vi "SpectrumIndex.vi"(9 "Freq":dbl=867920000.0 format="%#_13g", 11 "Spectrum":cluster{"f0":dbl, "df":dbl, "magnitude":dbl[]}) -> (1 "magnitude":dbl)   [LabVIEW 2020]
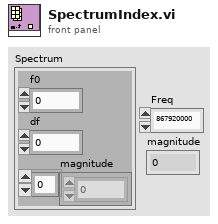
[diagram p1: front panel]
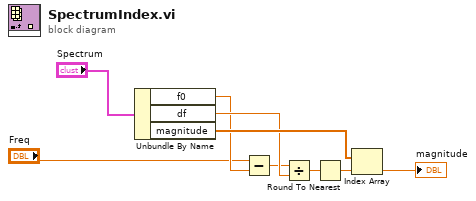
[diagram p0: block diagram]
diagram:
  n1 = Unbundle By Name("Spectrum") -> ("f0"=w3:dbl, "df"=w5:dbl, "magnitude"=w8:dbl[])
  n2 = Subtract(x="Freq", y=w3) -> (x-y=w4:dbl)
  n3 = Divide(x=w4, y=w5) -> (x/y=w6:dbl)
  n4 = Round To Nearest(number=w6) -> (nearest integer value=w7:dbl)
  n5 = Index Array(array=w8, index=w7) -> (element=→"magnitude":dbl)
